vi "Get Core Channel Settings.vi"(8 "error in (no error)":errorcluster, 11 "Item Ref in":T3 format="%.0x") -> (0 "error out":errorcluster, 2 "channel configuration":T1={"name"="Channel", "units"="V", "engine data type"=enum."DBL", "string data type"=enum."DBL", "string offset"=0} {"string offset" format="%d bytes"}, 3 "Item Ref out":T3 format="%.0x")   [LabVIEW 2017, in "DSF Shared.lvlib"]
uses:
  DSF Shared.lvlib
  <vilib>/NI Veristand/Custom Device API/Custom Device Item Ref.ctl
  DSF Core.lvlibp/Typedefs/Core Channel Configuration.ctl
  DSF Core.lvlibp/Typedefs/DSF Data Type.ctl
  <vilib>/NI Veristand/Custom Device API/Get Item Property (Variant).vi
  <vilib>/NI Veristand/Custom Device API/Custom Device API.lvlib
  DSF Core.lvlibp
  DSF Core.lvlibp/Classes/Configuration/Core/Channel/Channel Configuration.lvclass
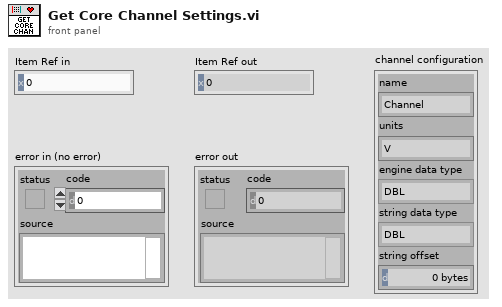
[diagram p1: front panel]
types:
  T1 = typedef "DSF Core.lvlibp/Channel Configuration.lvclass/Core Channel Configuration.ctl" = cluster{"name":string, "units":string, "engine data type":T2, "string data type":T2, "string offset":u64}
  T2 = typedef "DSF Core.lvlibp/DSF Data Type.ctl" = enum8{"Bool", "SGL", "DBL", "I8", "I16", "I32", "I64", "U8", "U16", "U32", "U64"}
  T3 = typedef "Custom Device API.lvlib/Custom Device Item Ref.ctl" = u64
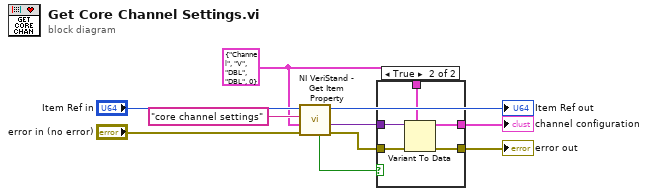
[diagram p0: block diagram]
diagram:
  w1 = T1 {"name"="Channel", "units"="V", "engine data type"=enum."DBL", "string data type"=enum."DBL", "string offset"=0} ("channel configuration")
  n1 = call-poly <vilib>:"NI VeriStand - Get Item Property.vi"("error in (no error)"="error in (no error)", "Default Value"=w1, "Property Name"="core channel settings" ("dsf options"), "Item Ref in"="Item Ref in") -> ("error out"=w9:errorcluster, "Value"=w8:variant, "Item Ref out"=→"Item Ref out":T3, "Found?"=w5:bool)  [unwired: 4 in]
  n2 = case shown="True" w5 {
    tunnel: w9 -> [w11 w17]
    tunnel: w1 -> [w12 w16]
    tunnel: w8 -> [_ w15]
    tunnel: [w11 w14] -> w7
    tunnel: [w12 w13] -> w4
    frame False {
    }
    frame True {
      n3 = Variant To Data(error in=w17, type=w16, Variant=w15) -> (data=w13:T1, error out=w14:errorcluster)
    }
  }
  "error out" <- w7
  "channel configuration" <- w4
